vi "GetLimitExpression.vi"(8 "error in":errorcluster, 11 "MeasureLimit in":refnum<class "MeasureLimit.lvclass">) -> (0 "error out":errorcluster, 2 "LimitExpression":string, 3 "MeasureLimit out":refnum<class "MeasureLimit.lvclass">)   [LabVIEW 2021, in "ProligentXMLGenerator.lvlib" / "MeasureLimit.lvclass"]
doc: "Defines the numeric precision of the measure value."
uses:
  MeasureLimit.lvclass
  MeasureLimit.lvclass/MeasureLimit.ctl
  Base/NonEmptyString_2000/NonEmptyString_2000.lvclass
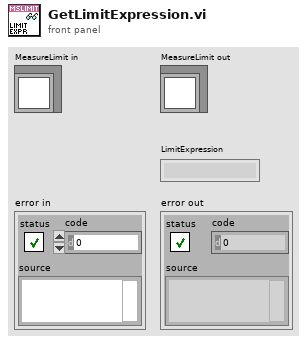
[diagram p1: front panel]
types:
  T1 = typedef "ProligentXMLGenerator.lvlib/MeasureLimit.lvclass/Data.ctl" = cluster{"Name":string, "CustomData":refnum<class "CustomData.lvclass">, "LimitExpression":refnum<class "NonEmptyString_2000.lvclass">}
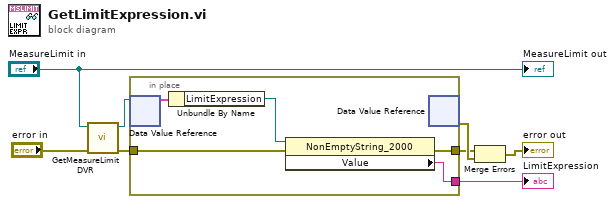
[diagram p0: block diagram]
diagram:
  n1 = call "GetMeasureLimitDVR.vi"("error in"="error in", "MeasureLimit"="MeasureLimit in") -> ("error out"=w2:errorcluster, "DVRReference"=w7:refnum<data-value>)  [unwired: 8 in]
  n2 = in-place "In Place Element Structure" {
    in-place-border: [w12] -> w6
    in-place-border: w2 -> [w9]
    in-place-border: [w11] -> w1
    n3 = in-place-dvr #1(w7) -> (w13:T1)  [unwired: 1 out]
    n4 = Unbundle By Name(w13) -> ("LimitExpression"=w10:refnum<class "NonEmptyString_2000.lvclass">)
    n5 = property on="Property Node" class="NonEmptyString_2000"(reference=w10, error in=w9) -> (error out=w11:errorcluster, "Value"=w12:string)  [unwired: 1 out]
    n6 = in-place-dvr #1() -> (w8:errorcluster)  [unwired: 1 in, 1 out]
  }
  "LimitExpression" <- w6
  n7 = Merge Errors(w1, w8) -> (→"error out":errorcluster)
  "MeasureLimit out" <- "MeasureLimit in"
